vi "ExDriver.vi"(4 "Error In":errorcluster, 7 "Command":string) -> (0 "Error Out":errorcluster, 3 "Response":string)   [LabVIEW 2018]
uses:
  MOKO_LabViewLibrary/MokoLowLevel/MokoLowLovelControl/MLLC_DriverName.ctl
  MOKO_LabViewLibrary/MokoLowLevel/MokoLowLovelControl/MLLC_DriverConnectCluster.ctl
  MOKO_LabViewLibrary/MokoLowLevel/MokoLowLovelControl/MLLC_InterfaceType.ctl
  MOKO_LabViewLibrary/MokoLowLevel/MokoLowLovelControl/MLLC_OpenedSession.ctl
  MOKO_LabViewLibrary/MokoLowLevel/MokoLowLovelControl/MLLC_InterfaceSettings.ctl
  MOKO_LabViewLibrary/MokoLowLevel/MokoLowLovelControl/MLLC_InterfaceKind.ctl
  MOKO_LabViewLibrary/MokoLowLevel/MokoLowLovelControl/MLLC_Request.ctl
  MOKO_LabViewLibrary/MokoLowLevel/MokoLowLovelControl/MLLC_ResponseInit.ctl
panel:
  in  "Response Init":T1="43B"
  in  "Request":T2="ID"
  in  "DriverSettings":T8={"DriverConnect"={"InterfaceType"=enum."VISA", "OpenedSession"="", "InterfaceSettings"={"Interface"=enum."RS232", "EOS 4 read"=enum."LF (\\n)", "EOS 4 write"=enum."LF (\\n)", "TMO, ms"=10000, "Sett"=variant(cluster{"Baud Rate":u32, "Data Bits":u16, "Parity":u16, "Stop Bits":u16, "Flow Control":u16, "Eho":bool} {"Baud Rate"=75, "Data Bits"=0, "Parity"=0, "Stop Bits"=0, "Flow Control"=0, "Eho"=FALSE})}}, "Values"={"Value"=0.0}}
  in  "Error Code":u32
  in  "Driver Name":T9="ExDriver"
  in  "Mode":T10(ring)
  # "ExDriver"
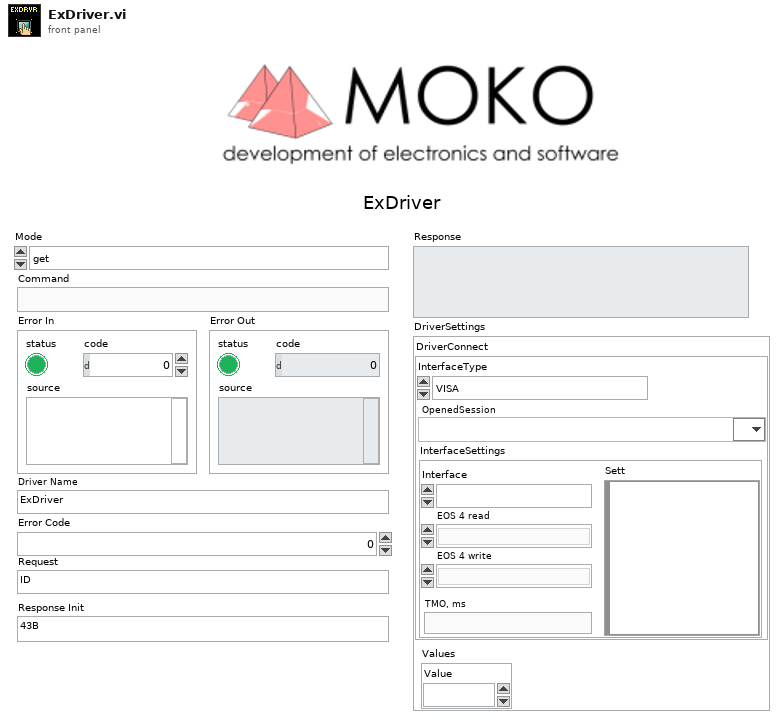
[diagram p1: front panel]
types:
  T1 = typedef "MLLC_ResponseInit.ctl" = string
  T2 = typedef "MLLC_Request.ctl" = string
  T3 = typedef "MLLC_DriverConnectCluster.ctl" = cluster{"InterfaceType":T4, "OpenedSession":T5, "InterfaceSettings":T6}
  T4 = typedef "MLLC_InterfaceType.ctl" = enum16{"VISA", "Prologix USB-GPIB"}
  T5 = typedef "MLLC_OpenedSession.ctl" = refnum<visa-resource-name>
  T6 = typedef "MLLC_InterfaceSettings.ctl" = cluster{"Interface":T7, "EOS 4 read":enum16{"Default (=EOS 4 write)", "CR (\\r)", "LF (\\n)", "None"}, "EOS 4 write":enum16{"CR+LF (\\r\\n)", "CR (\\r)", "LF (\\n)", "None"}, "TMO, ms":i32, "Sett":variant}
  T7 = typedef "MLLC_InterfaceKind.ctl" = enum16{"RS232", "GPIB", "USB", "Ethernet", "another"}
  T8 = cluster{"DriverConnect":T3, "Values":cluster{"Value":dbl}}
  T9 = typedef "MLLC_DriverName.ctl" = string
  T10 = enum16{"get", "set", "close", "Init", "Check", "ID"}
  T11 = typedef "MLLC_Mode.ctl" = enum16{"get", "set", "close", "Init", "Check"}
  T12 = typedef "MLLC_Error.ctl" = errorcluster
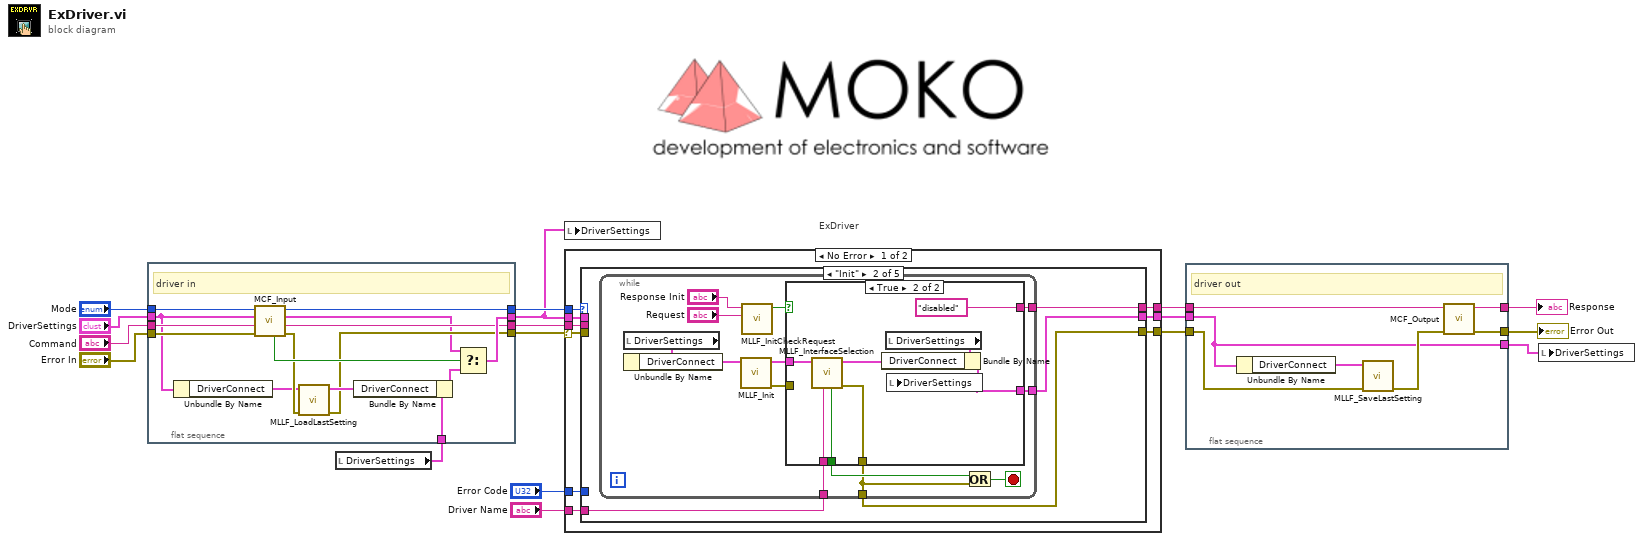
[diagram p0: block diagram]
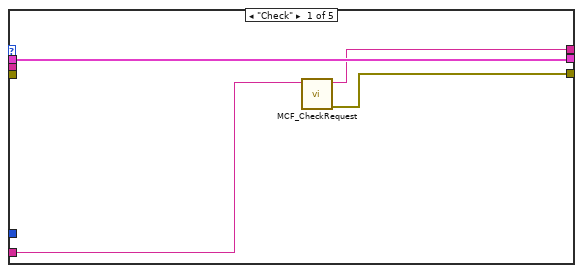
[diagram p2: hidden frame]
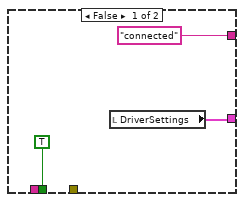
[diagram p3: hidden frame]
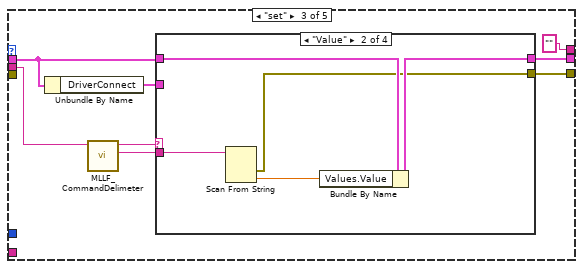
[diagram p4: hidden frame]
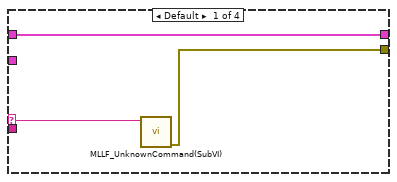
[diagram p5: hidden frame]
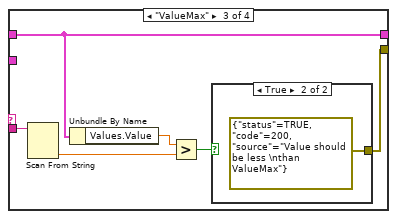
[diagram p6: hidden frame]
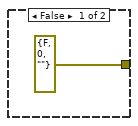
[diagram p7: hidden frame]
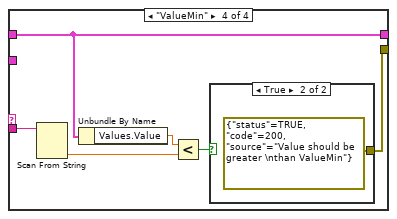
[diagram p8: hidden frame]
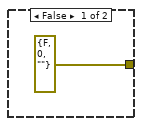
[diagram p9: hidden frame]
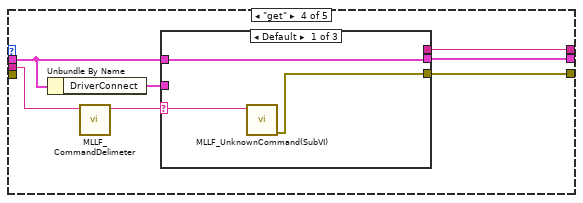
[diagram p10: hidden frame]
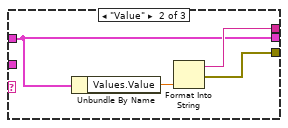
[diagram p11: hidden frame]
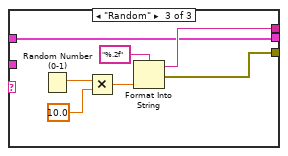
[diagram p12: hidden frame]
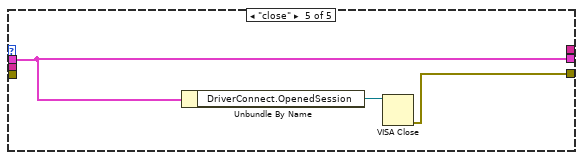
[diagram p13: hidden frame]
diagram:
  # "ExDriver"
  n1 = flat-sequence {
    tunnel: [w22] -> w8
    tunnel: [w24] -> w7
    tunnel: "Command" -> [w25]
    tunnel: "Mode" -> [w27]
    tunnel: "DriverSettings" -> [w19]
    tunnel: [w29] -> w10
    tunnel: w9 -> [w28]
    tunnel: "Error In" -> [w21]
    tunnel: [w20] -> w11
    frame #0 {
      # "driver in"
      n2 = Unbundle By Name(w19) -> ("DriverConnect"=w18:T3)
      n3 = call "MCF_Input.vi"("error in (no error)"=w21, "Command"=w25, "Mode"=w27) -> ("error out"=w23:errorcluster, "Command out"=w24:string, "Mode out"=w20:T11, "Boolean"=w26:bool)  [unwired: 5 in]
      n4 = call "MLLF_LoadLastSetting.vi"("Error In"=w23, "DriverConnectCluster in"=w18) -> ("Error Out"=w22:errorcluster, "DriverConnectCluster out"=w30:T3)  [unwired: 8 in]
      n5 = Bundle By Name(cluster=w28, "DriverConnect"=w30) -> (w31:T8)
      n6 = Select(t=w19, s=w26, f=w31) -> (s? t:f=w29:T8)
    }
  }
  n7 = local read "DriverSettings"() -> (w9:T8)
  n8 = local write "DriverSettings"(w10) -> ()
  n9 = case shown="No Error" w8 {
    selector: w8 -> [w36 w130]
    tunnel: [w38 w130] -> w4
    tunnel: w11 -> [w40 _]
    tunnel: [w39 _] -> w6
    tunnel: w7 -> [w37 _]
    tunnel: w10 -> [w33 w129]
    tunnel: "Error Code" -> [w35 _]
    tunnel: "Driver Name" -> [w34 _]
    tunnel: [w32 w129] -> w5
    frame No Error {
      n10 = case shown="\"Init\"" w40 {
        tunnel: [w42 w46 "" ("Output String") w105 _] -> w39
        tunnel: [w41 w48 w73 w106 w127] -> w38
        tunnel: w37 -> [_ _ w76 w108 _]
        tunnel: w36 -> [_ _ _ _ _]
        tunnel: w35 -> [_ _ _ _ _]
        tunnel: w34 -> [w43 w45 _ _ _]
        tunnel: w33 -> [w44 _ w80 w111 w126]
        tunnel: [w44 w47 w79 w110 w126] -> w32
        frame "Check" {
          # "Проверка подленности пользователя в соответствии с протоколом MD5."
          n11 = call "MCF_CheckRequest.vi"("Driver Name"=w43) -> ("Error Out"=w41:errorcluster, "Output String"=w42:string)  [unwired: 9 in]
        }
        frame "Init" {
          # "Тут проходит инициализация оборудования"
          n12 = while {
            tunnel: [w60] -> w48
            tunnel: w45 -> [w53]
            tunnel: [w57] -> w47
            tunnel: [w54] -> w46
            stop <- w59 stop-if-true
            n13 = local read "DriverSettings"() -> (w58:T8)
            n14 = Unbundle By Name(w58) -> ("DriverConnect"=w56:T3)
            n15 = call "MLLF_Init.vi"("DriverConnect in"=w56) -> ("Error Out"=w49:errorcluster, "DriverConnect out"=w55:T3)  [unwired: 7 in]
            n16 = call "MLLF_InitCheckRequest.vi"("Answer"="Request", "Response Init"="Response Init") -> ("Design"=w50:bool)  [unwired: 8 in, 1 out]
            n17 = case shown="True" w50 {
              tunnel: w55 -> [_ w71]
              tunnel: [TRUE w67] -> w61
              tunnel: [_ w72] -> w60
              tunnel: [w63 w68] -> w57
              tunnel: ["connected" "disabled"] -> w54
              tunnel: w53 -> [_ w65]
              tunnel: w49 -> [_ _]
              frame False {
                n18 = local read "DriverSettings"() -> (w63:T8)
              }
              frame True {
                n19 = call "MLLF_InterfaceSelection.vi"("Driver Name"=w65, "DriverConnect in"=w71) -> ("error out"=w72:T12, "DriverConnect out"=w70:T3, "stop init?"=w67:bool)  [unwired: 7 in]
                n20 = local read "DriverSettings"() -> (w69:T8)
                n21 = Bundle By Name(cluster=w69, "DriverConnect"=w70) -> (w68:T8)
                n22 = local write "DriverSettings"(w68) -> ()
              }
            }
            n23 = Or(x=w61, y=w60) -> (x .or. y?=w59:bool)
          }
        }
        frame "set" {
          # "Тут реализованы функции DriverSet"
          n24 = Unbundle By Name(w80) -> ("DriverConnect"=w77:T3)
          n25 = call "MLLF_CommandDelimeter.vi"("command with param"=w76) -> ("param 1"=w74:string, "command"=w75:string)  [unwired: 7 in, 2 out]
          n26 = case shown="\"Value\"" w75 {
            selector: w75 -> [w82 _ _ _]
            tunnel: [w83 w85 w89 w97] -> w79
            tunnel: w80 -> [w83 w88 w89 w97]
            tunnel: w77 -> [_ _ _ _]
            tunnel: w74 -> [_ w87 w94 w102]
            tunnel: [w81 w84 w90 w98] -> w73
            frame Default {
              n27 = call "MLLF_UnknownCommand(SubVI).vi"("Unknown command"=w82) -> ("error out"=w81:errorcluster)  [unwired: 10 in]
            }
            frame "Value" {
              n28 = Scan From String(input string=w87) -> (error out=w84:errorcluster, output 1=w86:dbl)  [unwired: 4 in, 2 out]
              n29 = Bundle By Name(cluster=w88, "Values.Value"=w86) -> (w85:T8)
            }
            frame "ValueMax" {
              n30 = Scan From String(input string=w94) -> (output 1=w93:dbl)  [unwired: 4 in, 3 out]
              n31 = Unbundle By Name(w89) -> ("Values.Value"=w92:dbl)
              n32 = Greater?(x=w92, y=w93) -> (0:w91:bool)
              n33 = case shown="True" w91 {
                tunnel: [errorcluster {"status"=FALSE, "code"=0, "source"=""} ("error IO") errorcluster {"status"=TRUE, "code"=200, "source"="Value should be less \nthan ValueMax"} ("error IO")] -> w90
                frame False {
                }
                frame True {
                }
              }
            }
            frame "ValueMin" {
              n34 = Scan From String(input string=w102) -> (output 1=w101:dbl)  [unwired: 4 in, 3 out]
              n35 = Unbundle By Name(w97) -> ("Values.Value"=w100:dbl)
              n36 = Less?(x=w100, y=w101) -> (x < y?=w99:bool)
              n37 = case shown="True" w99 {
                tunnel: [errorcluster {"status"=FALSE, "code"=0, "source"=""} ("error IO") errorcluster {"status"=TRUE, "code"=200, "source"="Value should be greater \nthan ValueMin"} ("error IO")] -> w98
                frame False {
                }
                frame True {
                }
              }
            }
          }
        }
        frame "get" {
          # "Тут реализованы функции DriverGet"
          n38 = Unbundle By Name(w111) -> ("DriverConnect"=w109:T3)
          n39 = call "MLLF_CommandDelimeter.vi"("command with param"=w108) -> ("command"=w107:string)  [unwired: 7 in, 3 out]
          n40 = case shown="Default" w107 {
            selector: w107 -> [w113 _ _]
            tunnel: w109 -> [_ _ _]
            tunnel: w111 -> [w114 w116 w124]
            tunnel: [w114 w116 w124] -> w110
            tunnel: [w112 w115 w119] -> w106
            tunnel: [_ w117 w125] -> w105
            frame Default {
              n41 = call "MLLF_UnknownCommand(SubVI).vi"("Unknown command"=w113) -> ("error out"=w112:errorcluster)  [unwired: 10 in]
            }
            frame "Value" {
              n42 = Unbundle By Name(w116) -> ("Values.Value"=w118:dbl)
              n43 = Format Into String(w118) -> (resulting string=w117:string, error out=w115:errorcluster)  [unwired: 3 in]
            }
            frame "Random" {
              n44 = Random Number (0-1)() -> (number: 0 to 1=w123:dbl)
              n45 = Multiply(x=w123, y=10.0) -> (x*y=w121:dbl)
              n46 = Format Into String(format string="%.2f", w121) -> (resulting string=w125:string, error out=w119:errorcluster)  [unwired: 2 in]
            }
          }
        }
        frame "close" {
          # "Завершение сессии"
          n47 = Unbundle By Name(w126) -> ("DriverConnect.OpenedSession"=w128:T5)
          n48 = VISA Close(VISA resource name=w128) -> (error out=w127:errorcluster)  [unwired: 1 in]
        }
      }
    }
    frame Error {
    }
  }
  n49 = flat-sequence {
    tunnel: [w137] -> w3
    tunnel: w6 -> [w136]
    tunnel: w4 -> [w131]
    tunnel: w5 -> [w132]
    tunnel: [w132] -> w1
    tunnel: [w133] -> w2
    frame #0 {
      # "driver out"
      n50 = Unbundle By Name(w132) -> ("DriverConnect"=w135:T3)
      n51 = call "MLLF_SaveLastSetting.vi"("error in"=w131, "DriverConnectCluster in"=w135) -> ("error out"=w134:T12)  [unwired: 8 in, 1 out]
      n52 = call "MCF_Output.vi"("Error In"=w134, "Input"=w136) -> ("Error Out"=w133:errorcluster, "Output"=w137:string)  [unwired: 8 in]
    }
  }
  n53 = local write "DriverSettings"(w1) -> ()
  "Response" <- w3
  "Error Out" <- w2
